vi "Actor Core.vi"(8 "error in":errorcluster, 11 "Machine d'état in":refnum<class "Machine d'état.lvclass">) -> (0 "error out":errorcluster, 3 "Actor out":refnum<class "Actor.lvclass">)   [LabVIEW 2020, in "Machine d'état.lvlib" / "Machine d'état.lvclass"]
doc: "(<B>Filename</B>: Actor Framework.lvlib:Actor.lvclass:Actor Core.vi)\n\nReceives messages to the actor, reacts to them, and initiates any error handling that may shut the actor down.\n\nDescendant classes may override this VI to append parallel tasks for the actor to complete while it handles messages. Overrides use the Call Parent Class Method node."
uses:
  C:/Program Files/National Instruments/LabVIEW 2020/vi.lib/ActorFramework/Actor/Actor.lvclass
  <vilib>/ActorFramework/Actor/Actor.lvclass
  <vilib>/ActorFramework/Actor/Actor.lvclass/Actor.ctl
  <vilib>/ActorFramework/Message Enqueuer/Message Enqueuer.lvclass/Message Enqueuer.ctl
  <vilib>/ActorFramework/Message Enqueuer/Init from Existing Queue.vi
  <vilib>/ActorFramework/Message Enqueuer/Enqueue.vi
  C:/Program Files/National Instruments/LabVIEW 2020/vi.lib/ActorFramework/Message/Message.lvclass
  <vilib>/ActorFramework/Stop Msg/Stop Msg.lvclass
  <vilib>/ActorFramework/Message Priority Queue/Priority Enqueue.vi
  <vilib>/ActorFramework/Message Enqueuer/Message Enqueuer.lvclass
panel:
  in  "Btn_Error":bool
  in  "Btn_Send":bool
  in  "Message":string
  out "Counter":u8
  in  "Btn_2":bool
  in  "Btn_1":bool
  out "Display":string
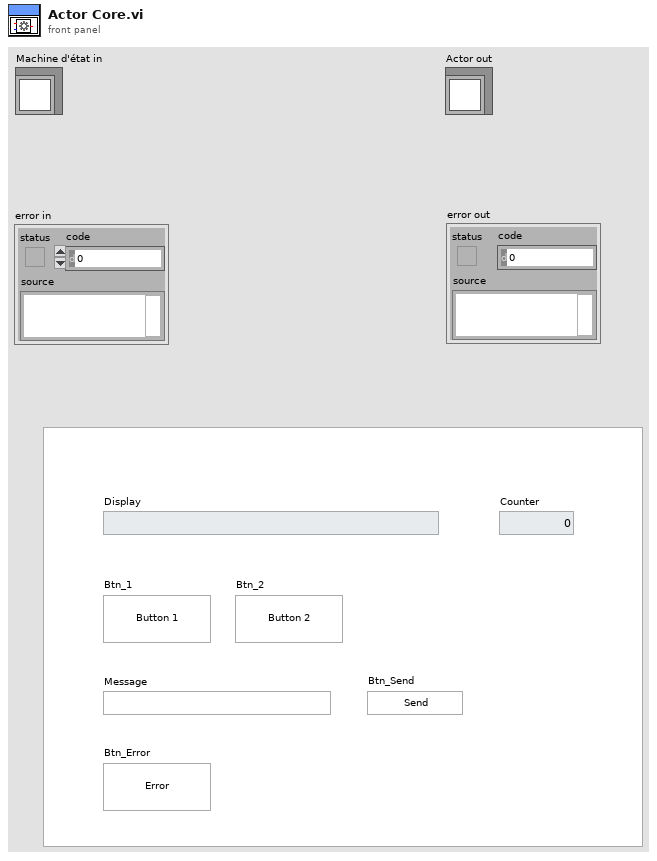
[diagram p1: front panel]
types:
  T1 = cluster{"Quit":refnum<user-event>, "Display":refnum<user-event>}
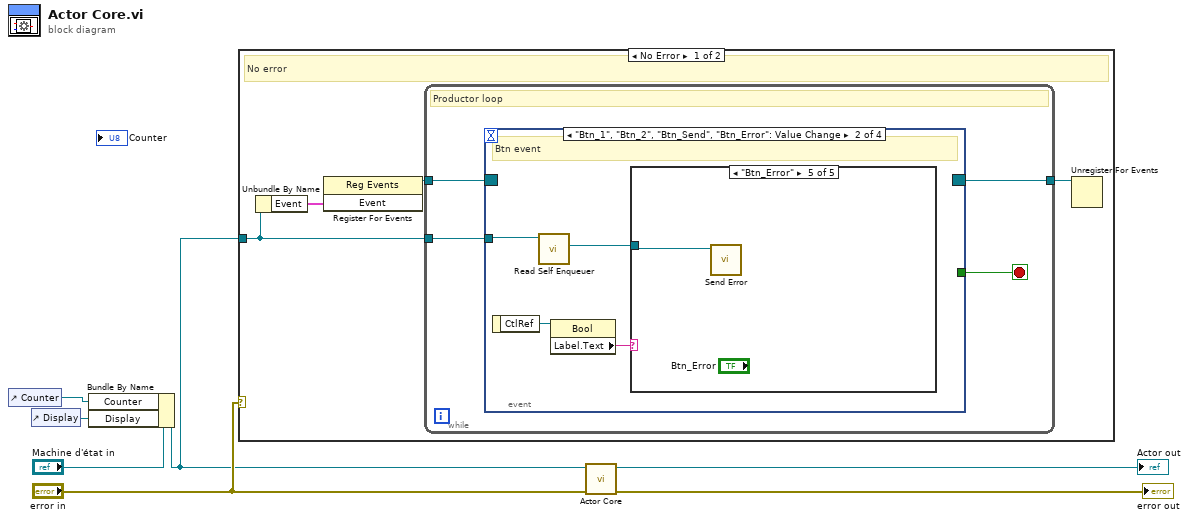
[diagram p0: block diagram]
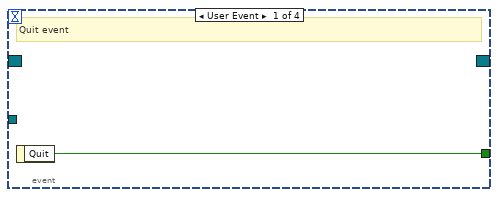
[diagram p2: hidden frame]
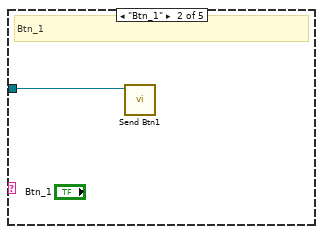
[diagram p4: hidden frame]
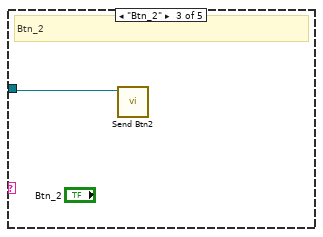
[diagram p5: hidden frame]
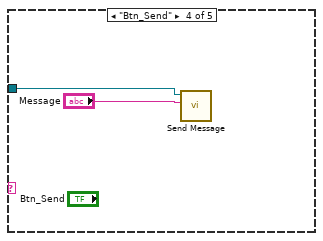
[diagram p6: hidden frame]
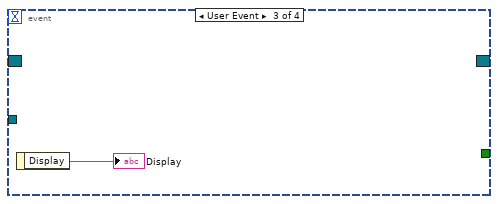
[diagram p7: hidden frame]
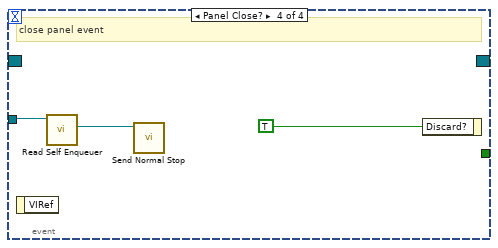
[diagram p8: hidden frame]
diagram:
  n1 = control-ref of="Counter"() -> (w1:refnum<vi>)
  n2 = control-ref of="Display"() -> (w2:refnum<vi>)
  n3 = Bundle By Name(cluster="Machine d'état in", "Counter"=w1, "Display"=w2) -> (w3:refnum<class "Machine d'état.lvclass">)
  n4 = case shown="No Error" "error in" {
    tunnel: w3 -> [w11 _]
    frame No Error {
      # "No error"
      n5 = Unbundle By Name(w11) -> ("Event"=w10:T1)
      n6 = register-events(w10) -> (reference out=w9:refnum<event-registration>)  [unwired: 2 in, 1 out]
      n7 = while {
        tunnel: w11 -> [w12]
        tunnel: w9 -> [w15]
        tunnel: [w13] -> w8
        stop <- w14 stop-if-true
        # "Productor loop"
        n8 = event shown="[1] \"Btn_1\", \"Btn_2\", \"Btn_Send\", \"Btn_Error\": Value Change" {
          selector: w15 -> [_ _ _ _]
          dyn-events: [_ _ _ _] -> w13
          timeout: _ -> [_ _ _ _]
          tunnel: [w16 _ _ _] -> w14
          tunnel: w12 -> [_ w18 _ w28]
          event User Event {
            # "Quit event"
            n9 = event-data() -> ("Quit"=w16:bool)  [unwired: 1 in]
          }
          event "Btn_1", "Btn_2", "Btn_Send", "Btn_Error": Value Change {
            # "Btn event"
            n10 = event-data() -> ("CtlRef"=w20:refnum<vi>)  [unwired: 1 in]
            n11 = call <vilib>:"Read Self Enqueuer.vi"("Actor"=w18) -> ("Self Enqueuer"=w17:refnum<class "Message Enqueuer.lvclass">)  [unwired: 10 in]
            n12 = property class="Bool"(reference=w20) -> ("Label.Text"=w19:string)  [unwired: 1 in, 2 out]
            n13 = case shown="\"Btn_Error\"" w19 {
              tunnel: w17 -> [_ w21 w22 w24 w25]
              frame Default {
                # "Default"
              }
              frame "Btn_1" {
                # "Btn_1"
                n14 = call "Send Btn1.vi"("Message Enqueuer"=w21) -> ()  [unwired: 9 in, 2 out]
              }
              frame "Btn_2" {
                # "Btn_2"
                n15 = call "Send Btn2.vi"("Message Enqueuer"=w22) -> ()  [unwired: 9 in, 2 out]
              }
              frame "Btn_Send" {
                n16 = call "Send Message.vi"("Message"="Message", "Message Enqueuer"=w24) -> ()  [unwired: 8 in, 2 out]
              }
              frame "Btn_Error" {
                n17 = call "Send Error.vi"("Message Enqueuer"=w25) -> ()  [unwired: 9 in, 2 out]
              }
            }
          }
          event User Event {
            n18 = event-data() -> ("Display"=→"Display":string)  [unwired: 1 in]
          }
          event Panel Close? {
            # "close panel event"
            n19 = event-data() -> ()  [unwired: 1 in, 1 out]
            n20 = call <vilib>:"Read Self Enqueuer.vi"("Actor"=w28) -> ("Self Enqueuer"=w27:refnum<class "Message Enqueuer.lvclass">)  [unwired: 10 in]
            n21 = call <vilib>:"Send Normal Stop.vi"("Message Enqueuer"=w27) -> ()  [unwired: 10 in, 1 out]
            n22 = event-data("Discard?"=TRUE) -> ()  [unwired: 1 in, 1 out]
          }
        }
      }
      n23 = Unregister For Events(event registration refnum=w8) -> ()  [unwired: 1 in, 1 out]
    }
    frame Error {
    }
  }
  n24 = call-parent "Actor Core.vi"("error in"="error in", "Actor in"=w3) -> ("error out"=→"error out":errorcluster, "Actor out"=→"Actor out":refnum<class "Actor.lvclass">)  [unwired: 8 in]
